vi "Report.vi"() -> ()   [LabVIEW 2017]
uses:
  <vilib>/Utility/miscctls.llb/LVRowAndColumnUnsignedTypeDef.ctl
  <vilib>/addons/database/Connection.llb/DB Tools Open Connec (String).vi
  <vilib>/Utility/file.llb/Write Delimited Spreadsheet (string).vi
  Global/Global 1.vi
  <vilib>/addons/database/NI_Database_API.lvlib
  <vilib>/Utility/NIReport.llb/NI_report.lvclass
  <vilib>/Utility/NIReport.llb/Append Text Table to Report (wrap).vi
panel:
  out "reposr save header":string[](array[string])
  out "subarray":string[](array[string])
  in  "SELECT REPORT TYPE":string(combo)="WITHOUT TRECIABILITY"
  out "error out":errorcluster
  in  "error in (no error)":errorcluster
  in  "GET REPORT":bool
  in  "EXIT":bool
  in  "EXPORT TO EXCEL":bool
  in  "TO":timestamp format="%<%x>T"
  in  "FROM":timestamp format="%<%x>T"
  in  "BARCODE":string
  in  "TYPE":string(combo)="DATE TIME"
  in  "STATION WISE":string(combo)="OP 10&20"
  out "Table":string[][](table)=[["16-06-2021 10:47:08", "A", "0.00", "0.00", "0.00", "2.03", "112.72", "3.22", "655.04", "OK"], ["16-06-2021 10:59:02", "A", "0.00", "0.00", "0.00", "0.00", "0.00", "3.02", "0.25", "NOK"]]
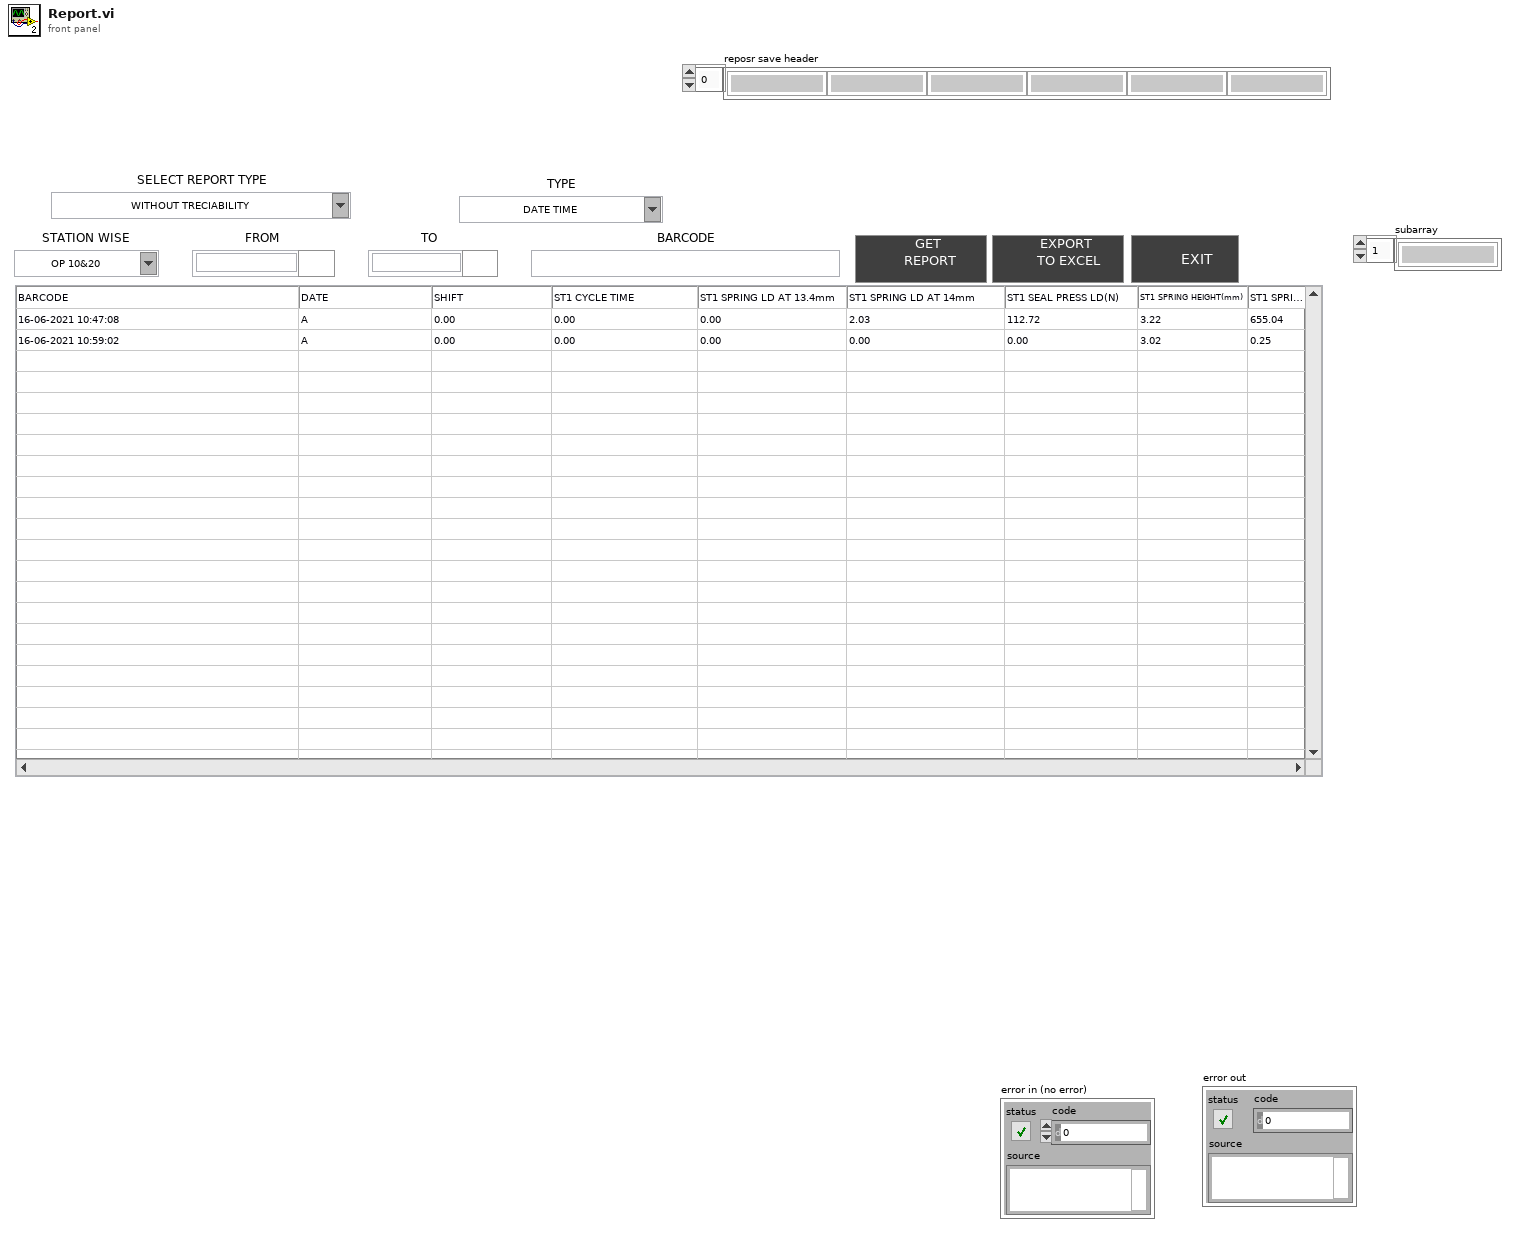
[diagram p1: front panel]
types:
  T1 = typedef "NI_Database_API.lvlib/Conn ObjectReference.ctl" = refnum<k1>
  T2 = typedef "LVRowAndColumnUnsignedTypeDef.ctl" = cluster{"Row":u32, "Column":u32}
  T3 = enum16{"Standard Report", "HTML", "Word", "Excel"}
  T4 = enum16{"maximized", "minimized", "normal", "no change"}
  T5 = enum32{"invalid app kind", "Development System", "Run Time System", "Student Edition", "Embedded LabVIEW", "Evaluation", "Custom"}
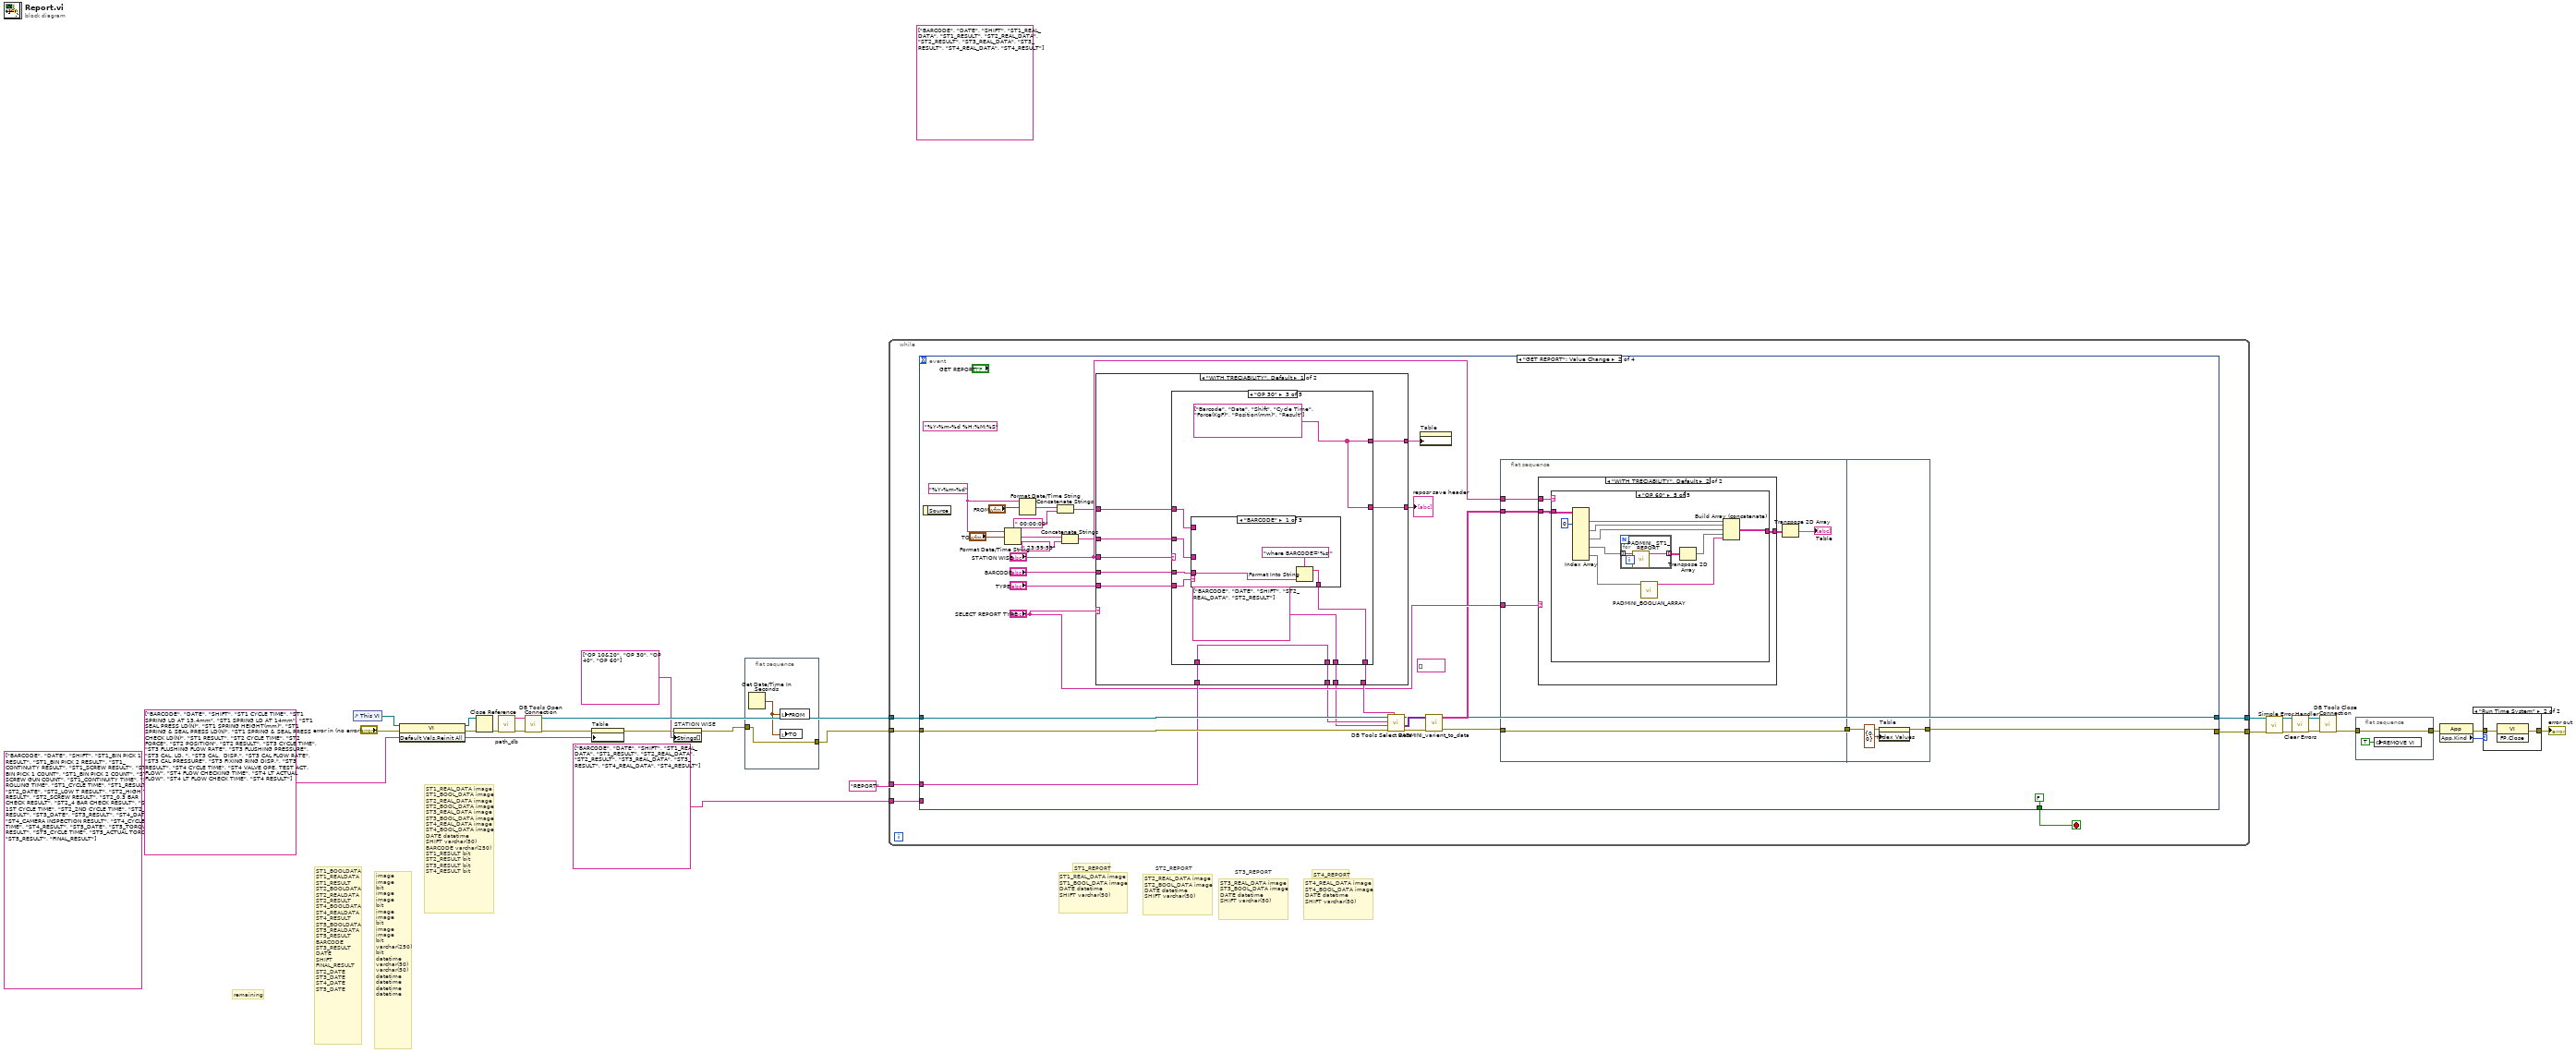
[diagram p0: block diagram]
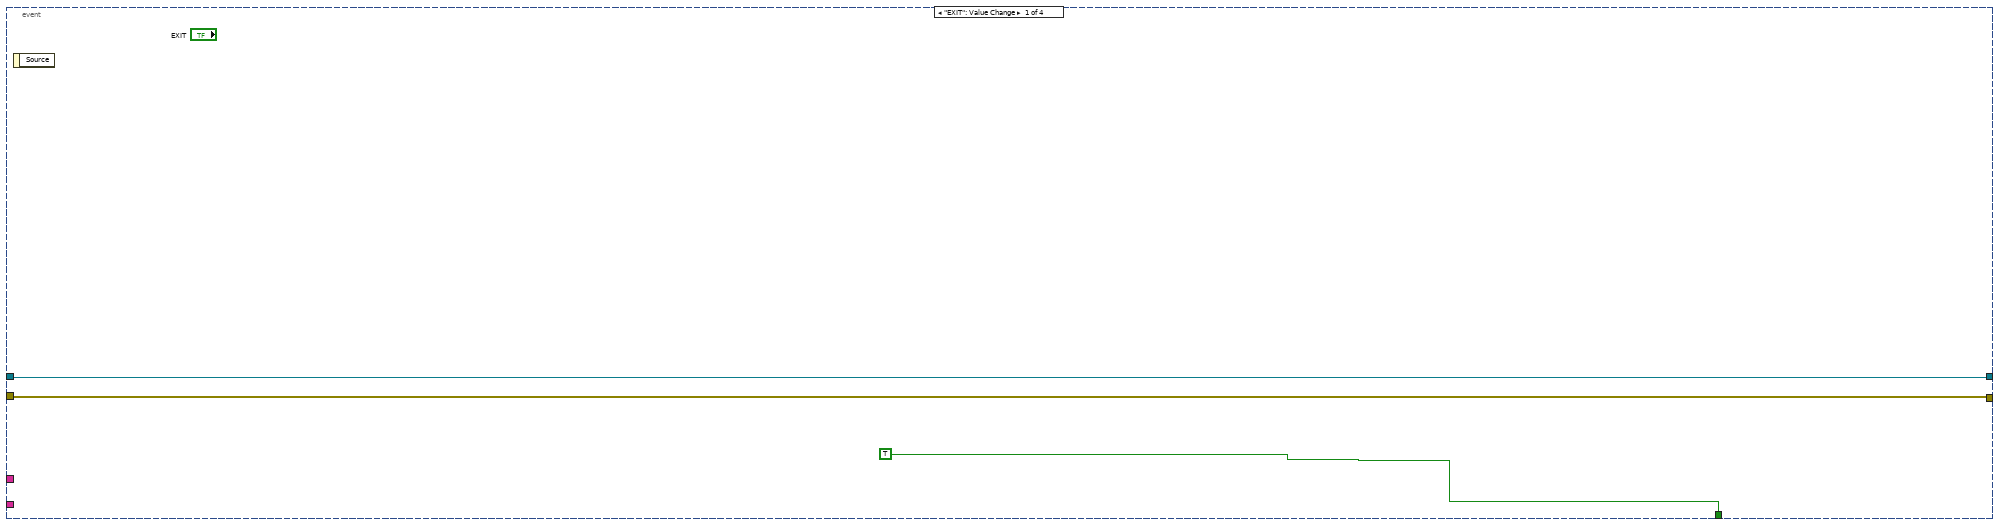
[diagram p2: hidden frame]
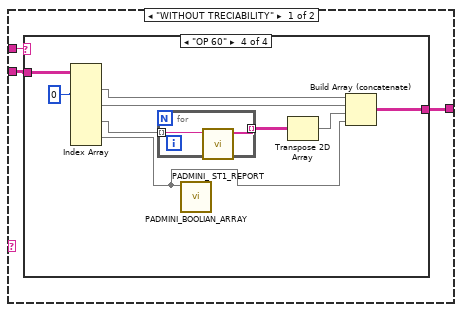
[diagram p3: hidden frame]
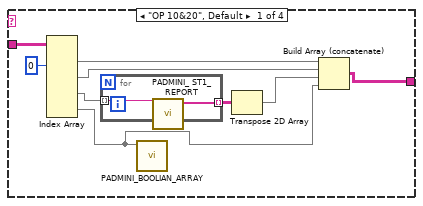
[diagram p4: hidden frame]
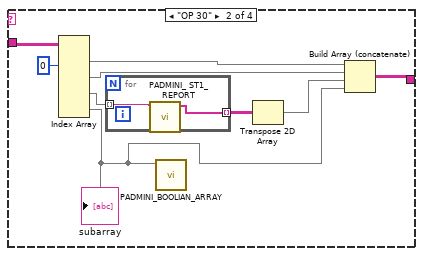
[diagram p5: hidden frame]
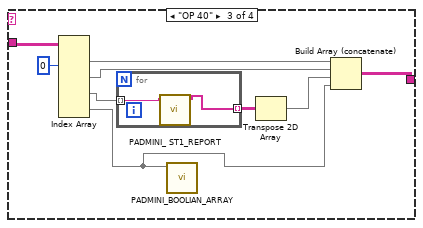
[diagram p6: hidden frame]
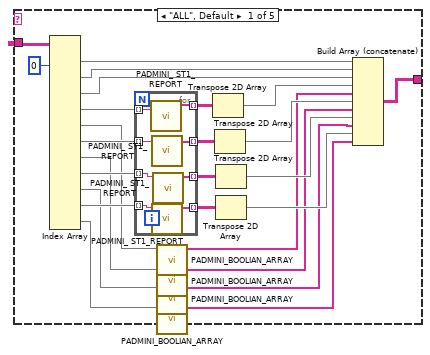
[diagram p7: hidden frame]
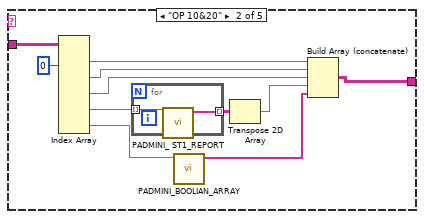
[diagram p8: hidden frame]
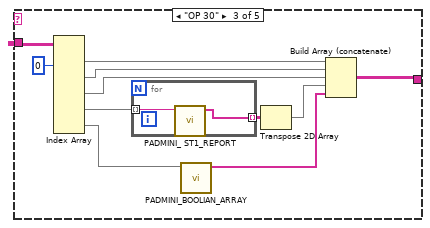
[diagram p9: hidden frame]
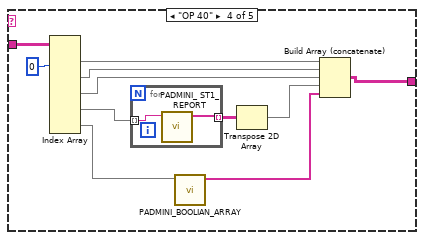
[diagram p10: hidden frame]
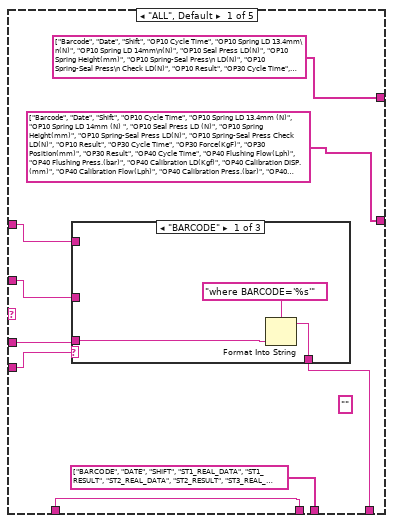
[diagram p11: hidden frame]
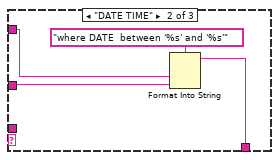
[diagram p12: hidden frame]
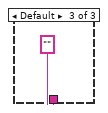
[diagram p13: hidden frame]
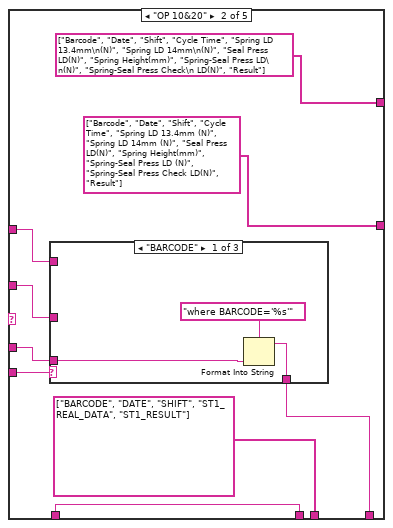
[diagram p14: hidden frame]
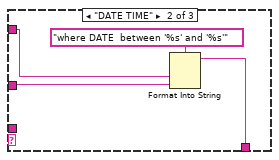
[diagram p15: hidden frame]
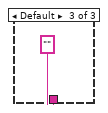
[diagram p16: hidden frame]
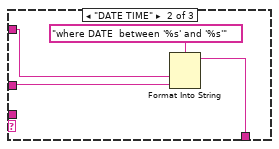
[diagram p17: hidden frame]
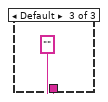
[diagram p18: hidden frame]
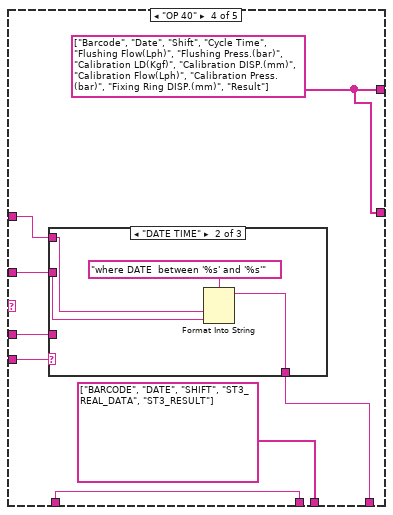
[diagram p19: hidden frame]
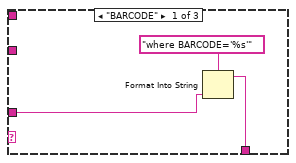
[diagram p20: hidden frame]
diagram:
  (unwired) string[] ["BARCODE", "DATE", "SHIFT", "ST1_REAL_DATA", "ST1_RESULT", "ST2_REAL_DATA", "ST2_RESULT", "ST3_REAL_DATA", "ST3_RESULT", "ST4_REAL_DATA", "ST4_RESULT"]
  (unwired) string[] ["BARCODE", "DATE", "SHIFT", "ST1_BIN PICK 1 RESULT", "ST1_BIN PICK 2 RESULT", "ST1_CONTINUITY RESULT", "ST1_SCREW RESULT", "ST1_BIN PICK 1 COUNT", "ST1_BIN PICK 2 COUNT", "ST1_SCREW GUN COUNT", "ST1_CONTINUITY TIME", "ST1_ROLLING TIME", "ST1_CYCLE TIME", "ST1_RESULT", "ST2_DATE", "ST2_LOW T RESULT", "ST2_HIGH T RESULT", "ST2_SCREW RESULT", "ST2_0.3 BAR CHECK RESULT", "ST2_4 BAR CHECK RESULT", "ST2_1ST CYCLE TIME", "ST2_2ND CYCLE TIME", "ST2_RESULT", "ST3_DATE", "ST3_RESULT", "ST4_DATE", "ST4_CAMERA INSPECTION RESULT", "ST4_CYCLE TIME", "ST4_RESULT", "ST5_DATE", "ST5_TORQUE RESULT", "ST5_CYCLE TIME", "ST5_ACTUAL TORQUE", "ST5_RESULT", "FINAL_RESULT"]
  # "remaining"
  # "ST4_REPORT"
  # "ST3_REPORT"
  # "ST2_REPORT"
  # "ST1_REPORT"
  # "ST4_REAL_DATA\timage\nST4_BOOL_DATA\timage\nDATE\tdatetime\nSHIFT\tvarchar(50)"
  # "ST3_REAL_DATA\timage\nST3_BOOL_DATA\timage\nDATE\tdatetime\nSHIFT\tvarchar(50)"
  # "ST2_REAL_DATA\timage\nST2_BOOL_DATA\timage\nDATE\tdatetime\nSHIFT\tvarchar(50)"
  # "ST1_REAL_DATA\timage\nST1_BOOL_DATA\timage\nDATE\tdatetime\nSHIFT\tvarchar(50)"
  # "ST1_REAL_DATA\timage\nST1_BOOL_DATA\timage\nST2_REAL_DATA\timage\nST2_BOOL_DATA\timage\nST3_REAL_DATA\timage\nST3_BOOL_DATA\timage\nST4_REAL_DATA\timage\nST4_BOOL_DATA\timage\nDATE\tdatetime\nSHIFT\tvarchar(50)\nBARCODE\tvarchar(250)\nST1_RESULT\tbit\nST2_RESULT\tbit\nST3_RESULT\tbit\nST4_RESULT\tbit"
  # "image\nimage\nbit\nimage\nimage\nbit\nimage\nimage\nbit\nimage\nimage\nbit\nvarchar(250)\nbit\ndatetime\nvarchar(50)\nvarchar(50)\ndatetime\ndatetime\ndatetime\ndatetime"
  # "ST1_BOOLDATA\nST1_REALDATA\nST1_RESULT\nST2_BOOLDATA\nST2_REALDATA\nST2_RESULT\nST4_BOOLDATA\nST4_REALDATA\nST4_RESULT\nST5_BOOLDATA\nST5_REALDATA\nST5_RESULT\nBARCODE\nST3_RESULT\nDATE\nSHIFT\nFINAL_RESULT\nST2_DATE\nST3_DATE\nST4_DATE\nST5_DATE"
  n1 = control-ref of="This VI"() -> (w25:refnum<vi>)
  n2 = invoke class="VI" method="Default Vals.Reinit All"(reference=w25, error in="error in (no error)") -> (reference out=w23:refnum<vi>, error out=w22:errorcluster)  [unwired: 1 in, 1 out]
  n3 = Close Reference(reference=w23, error in (no error)=w22) -> (error out=w12:errorcluster)
  n4 = call "path_db.vi"("error in"=w12) -> ("error out"=w14:errorcluster, "resulting string"=w13:string)  [unwired: 9 in]
  n5 = call-poly <vilib>:"DB Tools Open Connection.vi"("error in (no error)"=w14, "connection information"=w13) -> ("error out"=w6:errorcluster, "connection reference"=w11:T1)  [unwired: 6 in]
  n6 = property on="Table" class="Tbl (strict)"(error in=w6, "Column Headers[]"=string[] ["BARCODE", "DATE", "SHIFT", "ST1 CYCLE TIME", "ST1 SPRING LD AT 13.4mm", "ST1 SPRING LD AT 14mm", "ST1 SEAL PRESS LD(N)", "ST1 SPRING HEIGHT(mm)", "ST1 SPRING & SEAL PRESS LD(N)", "ST1 SPRING & SEAL PRESS CHECK LD(N)", "ST1 RESULT", "ST2 CYCLE TIME", "ST2 FORCE", "ST2 POSITION", "ST2 RESULT", "ST3 CYCLE TIME", "ST3 FLUSHING FLOW RATE", "ST3 FLUSHING PRESSURE", "ST3 CAL. LD. ", "ST3 CAL.  DISP.", "ST3 CAL FLOW RATE", "ST3 CAL PRESSURE", "ST3 FIXING RING DISP.", "ST3 RESULT", "ST4 CYCLE TIME", "ST4 VALVE OPE. TEST ACT. FLOW", "ST4 FLOW CHECKING TIME", "ST4 LT ACTUAL FLOW", "ST4 LT FLOW CHECK TIME", "ST4 RESULT"]) -> (error out=w3:errorcluster)  [unwired: 1 in, 1 out]
  n7 = property on="STATION WISE" class="CmbBox"(error in=w3, "Strings[]"=string[] ["OP 10&20", "OP 30", "OP 40", "OP 60"] ("Strings []")) -> (error out=w2:errorcluster)  [unwired: 1 in, 1 out]
  n8 = flat-sequence {
    tunnel: w2 -> [w26]
    tunnel: [w26] -> w1
    frame #0 {
      n9 = Get Date/Time In Seconds() -> (seconds since 1Jan1904=w27:timestamp)
      n10 = local write "FROM"(w27) -> ()
      n11 = local write "TO"(w27) -> ()
    }
  }
  n12 = while {
    tunnel: [w31] -> w15
    tunnel: w1 -> [w33]
    tunnel: w11 -> [w32]
    tunnel: [w30] -> w9
    tunnel: "REPORT" -> [w29]
    tunnel: string[] ["BARCODE", "DATE", "SHIFT", "ST1_REAL_DATA", "ST1_RESULT", "ST2_REAL_DATA", "ST2_RESULT", "ST3_REAL_DATA", "ST3_RESULT", "ST4_REAL_DATA", "ST4_RESULT"] -> [w28]
    stop <- w34 stop-if-true
    n13 = event shown="[1] \"GET REPORT\": Value Change" {
      selector: _ -> [_ _ _ _]
      dyn-events: _ -> [_ _ _ _]
      timeout: _ -> [_ _ _ _]
      tunnel: [TRUE FALSE FALSE FALSE] -> w34
      tunnel: w33 -> [w35 w65 w378 w389]
      tunnel: w32 -> [w36 w66 w381 w400]
      tunnel: [w36 w39 w381 w400] -> w30
      tunnel: [w35 w45 w377 w386] -> w31
      tunnel: w29 -> [_ w56 _ _]
      tunnel: w28 -> [_ _ _ _]
      event "EXIT": Value Change {
        n14 = event-data() -> ()  [unwired: 1 in, 1 out]
      }
      event "GET REPORT": Value Change {
        (unwired) string[] []
        (unwired) "%Y-%m-%d %H:%M:%S" ("time format string (%c)")
        w61 = "%Y-%m-%d" ("time format string (%c)")
        n15 = event-data() -> ()  [unwired: 1 in, 1 out]
        n16 = Format Date/Time String(time format string (%c)=w61, seconds (now)="TO") -> (date/time string=w50:string)  [unwired: 1 in]
        n17 = Format Date/Time String(time format string (%c)=w61, seconds (now)="FROM") -> (date/time string=w53:string)  [unwired: 1 in]
        n18 = Concatenate Strings(w53, " 00:00:00" ("time format string (%c)")) -> (w52:string)
        n19 = Concatenate Strings(w50, " 23:59:59" ("time format string (%c)")) -> (w49:string)
        n20 = case shown="\"WITH TRECIABILITY\", Default" "SELECT REPORT TYPE" {
          tunnel: "TYPE" -> [w222 w316]
          tunnel: [w221 w315] -> w63
          tunnel: "BARCODE" -> [w220 w314]
          tunnel: w52 -> [w219 w313]
          tunnel: w49 -> [w218 w312]
          tunnel: [w217 w311] -> w42
          tunnel: [w216 w310] -> w58
          tunnel: "STATION WISE" -> [w215 w309]
          tunnel: [w214 w308] -> w43
          tunnel: w56 -> [w213 w307]
          tunnel: [w212 w306] -> w44
          frame "WITH TRECIABILITY", Default {
            n21 = case shown="\"OP 30\"" w215 {
              tunnel: w222 -> [w225 w248 w264 w280 w297]
              tunnel: [w226 w247 w263 w279 w296] -> w221
              tunnel: w220 -> [w224 w246 w262 w278 w295]
              tunnel: w219 -> [w228 w245 w261 w277 w294]
              tunnel: w218 -> [w227 w244 w260 w276 w293]
              tunnel: [string[] ["BARCODE", "DATE", "SHIFT", "ST1_REAL_DATA", "ST1_RESULT", "ST2_REAL_DATA", "ST2_RESULT", "ST3_REAL_DATA", "ST3_RESULT", "ST4_REAL_DATA", "ST4_RESULT"] string[] ["BARCODE", "DATE", "SHIFT", "ST1_REAL_DATA", "ST1_RESULT"] string[] ["BARCODE", "DATE", "SHIFT", "ST2_REAL_DATA", "ST2_RESULT"] string[] ["BARCODE", "DATE", "SHIFT", "ST3_REAL_DATA", "ST3_RESULT"] string[] ["BARCODE", "DATE", "SHIFT", "ST4_REAL_DATA", "ST4_RESULT"]] -> w217
              tunnel: [string[] ["Barcode", "Date", "Shift", "OP10 Cycle Time", "OP10 Spring LD 13.4mm\n(N)", "OP10 Spring LD 14mm\n(N)", "OP10 Seal Press LD(N)", "OP10 Spring Height(mm)", "OP10 Spring-Seal Press\n LD(N)", "OP10 Spring-Seal Press\n Check LD(N)", "OP10 Result", "OP30 Cycle Time", "OP30 Force(KgF)", "OP30 Position(mm)", "OP30 Result", "OP40 Cycle Time", "OP40 Flushing Flow(Lph)", "OP40 Flushing Press.(bar)", "OP40 Calibration LD(Kgf)", "OP40 Calibration DISP.(mm)", "OP40 Calibration Flow(Lph)", "OP40 Calibration Press.(bar)", "OP40 Fixing Ring DISP.(mm)", "OP40 Result", "OP60 Cycle Time", "OP60 Valve Ope. Flow(Lpm)", "OP60 Pressure (Bar)", "OP60 Leat Test Flow(Ccm)", "OP60 LT Pressure (Bar)", "OP60 Result"] string[] ["Barcode", "Date", "Shift", "Cycle Time", "Spring LD 13.4mm\n(N)", "Spring LD 14mm\n(N)", "Seal Press LD(N)", "Spring Height(mm)", "Spring-Seal Press LD\n(N)", "Spring-Seal Press Check\n LD(N)", "Result"] w257 w273 string[] ["Barcode", "Date", "Shift", "Cycle Time", "Valve Ope. Flow(Lpm)", " Pressure (Bar)", "Leat Test Flow(Ccm)", "LT Pressure (Bar)", "Result"]] -> w216
              tunnel: [w231 w242 w258 w274 w291] -> w214
              tunnel: w213 -> [w231 w242 w258 w274 w291]
              tunnel: [string[] ["Barcode", "Date", "Shift", "OP10 Cycle Time", "OP10 Spring LD 13.4mm (N)", "OP10 Spring LD 14mm (N) ", "OP10 Seal Press LD (N)", "OP10 Spring Height(mm)", "OP10 Spring-Seal Press LD(N)", "OP10 Spring-Seal Press Check LD(N)", "OP10 Result", "OP30 Cycle Time", "OP30 Force(KgF)", "OP30 Position(mm)", "OP30 Result", "OP40 Cycle Time", "OP40 Flushing Flow(Lph)", "OP40 Flushing Press.(bar)", "OP40 Calibration LD(Kgf)", "OP40 Calibration DISP.(mm)", "OP40 Calibration Flow(Lph)", "OP40 Calibration Press.(bar)", "OP40 Fixing Ring DISP.(mm)", "OP40 Result", "OP60 Cycle Time", "OP60 Valve Ope. Flow(Lpm)", "OP60 Pressure (Bar)", "OP60 Leat Test Flow(Ccm)", "OP60 LT Pressure (Bar)", "OP60 Result"] string[] ["Barcode", "Date", "Shift", "Cycle Time", "Spring LD 13.4mm (N)", "Spring LD 14mm (N)", "Seal Press LD(N)", "Spring Height(mm)", "Spring-Seal Press LD (N)", "Spring-Seal Press Check LD(N)", "Result"] w257 w273 string[] ["Barcode", "Date", "Shift", "Cycle Time", "Valve Ope. Flow(Lpm)", "Pressure (Bar)", "Leat Test Flow(Ccm)", "LT Pressure (Bar)", "Result"]] -> w212
              frame "ALL", Default {
                (unwired) ""
                n22 = case shown="\"BARCODE\"" w225 {
                  tunnel: [w233 w237 ""] -> w226
                  tunnel: w224 -> [w232 _ _]
                  tunnel: w228 -> [_ w236 _]
                  tunnel: w227 -> [_ w235 _]
                  frame "BARCODE" {
                    n23 = Format Into String(format string="where BARCODE='%s'", w232) -> (resulting string=w233:string)  [unwired: 2 in, 1 out]
                  }
                  frame "DATE TIME" {
                    n24 = Format Into String(format string="where DATE  between '%s' and '%s'", w236, w235) -> (resulting string=w237:string)  [unwired: 2 in, 1 out]
                  }
                  frame Default {
                  }
                }
              }
              frame "OP 10&20" {
                n25 = case shown="\"BARCODE\"" w248 {
                  tunnel: [w250 w254 ""] -> w247
                  tunnel: w246 -> [w249 _ _]
                  tunnel: w245 -> [_ w253 _]
                  tunnel: w244 -> [_ w252 _]
                  frame "BARCODE" {
                    n26 = Format Into String(format string="where BARCODE='%s'", w249) -> (resulting string=w250:string)  [unwired: 2 in, 1 out]
                  }
                  frame "DATE TIME" {
                    n27 = Format Into String(format string="where DATE  between '%s' and '%s'", w253, w252) -> (resulting string=w254:string)  [unwired: 2 in, 1 out]
                  }
                  frame Default {
                  }
                }
              }
              frame "OP 30" {
                w257 = string[] ["Barcode", "Date", "Shift", "Cycle Time", "Force(KgF)", "Position(mm)", "Result"]
                n28 = case shown="\"BARCODE\"" w264 {
                  tunnel: [w266 w270 ""] -> w263
                  tunnel: w262 -> [w265 _ _]
                  tunnel: w261 -> [_ w269 _]
                  tunnel: w260 -> [_ w268 _]
                  frame "BARCODE" {
                    n29 = Format Into String(format string="where BARCODE='%s'", w265) -> (resulting string=w266:string)  [unwired: 2 in, 1 out]
                  }
                  frame "DATE TIME" {
                    n30 = Format Into String(format string="where DATE  between '%s' and '%s'", w269, w268) -> (resulting string=w270:string)  [unwired: 2 in, 1 out]
                  }
                  frame Default {
                  }
                }
              }
              frame "OP 40" {
                w273 = string[] ["Barcode", "Date", "Shift", "Cycle Time", "Flushing Flow(Lph)", "Flushing Press.(bar)", "Calibration LD(Kgf)", "Calibration DISP.(mm)", "Calibration Flow(Lph)", "Calibration Press.(bar)", "Fixing Ring DISP.(mm)", "Result"]
                n31 = case shown="\"DATE TIME\"" w280 {
                  tunnel: [w282 w286 ""] -> w279
                  tunnel: w278 -> [w281 _ _]
                  tunnel: w277 -> [_ w285 _]
                  tunnel: w276 -> [_ w284 _]
                  frame "BARCODE" {
                    n32 = Format Into String(format string="where BARCODE='%s'", w281) -> (resulting string=w282:string)  [unwired: 2 in, 1 out]
                  }
                  frame "DATE TIME" {
                    n33 = Format Into String(format string="where DATE  between '%s' and '%s'", w285, w284) -> (resulting string=w286:string)  [unwired: 2 in, 1 out]
                  }
                  frame Default {
                  }
                }
              }
              frame "OP 60" {
                n34 = case shown="\"DATE TIME\"" w297 {
                  tunnel: [w299 w303 ""] -> w296
                  tunnel: w295 -> [w298 _ _]
                  tunnel: w294 -> [_ w302 _]
                  tunnel: w293 -> [_ w301 _]
                  frame "BARCODE" {
                    n35 = Format Into String(format string="where BARCODE='%s'", w298) -> (resulting string=w299:string)  [unwired: 2 in, 1 out]
                  }
                  frame "DATE TIME" {
                    n36 = Format Into String(format string="where DATE  between '%s' and '%s'", w302, w301) -> (resulting string=w303:string)  [unwired: 2 in, 1 out]
                  }
                  frame Default {
                  }
                }
              }
            }
          }
          frame "WITHOUT TRECIABILITY" {
            n37 = case shown="\"OP 30\"" w309 {
              tunnel: w316 -> [w325 w338 w354 w367]
              tunnel: [w324 w337 w353 w366] -> w315
              tunnel: w314 -> [w323 w336 w352 w365]
              tunnel: w313 -> [w322 w335 w351 w364]
              tunnel: w312 -> [w321 w334 w350 w363]
              tunnel: [string[] ["DATE", "SHIFT", "ST1_REAL_DATA", "RESULT"] ("columns") string[] ["DATE", "SHIFT", "ST2_REAL_DATA", "RESULT"] string[] ["DATE", "SHIFT", "ST3_REAL_DATA", "RESULT"] string[] ["DATE", "SHIFT", "ST4_REAL_DATA", "RESULT"]] -> w311
              tunnel: [string[] ["Date", "Shift", "Cycle Time", "Spring LD 13.4mm\n(N)", "Spring LD 14mm\n(N)", "Seal Press LD(N)", "Spring Height(mm)", "Spring-Seal Press LD(N)", "Spring-Seal Press Check\n LD(N)", "Result"] w331 w347 w360] -> w310
              tunnel: ["ST1_REPORT" "ST2_REPORT" ("table") "ST3_REPORT" ("table") "ST4_REPORT" ("table")] -> w308
              tunnel: w307 -> [_ _ _ _]
              tunnel: [string[] ["Date", "Shift", "Cycle Time", "Spring LD 13.4mm (N)", "Spring LD 14mm (N)", "Seal Press LD(N)", "Spring Height(mm)", "Spring-Seal Press LD(N)", "Spring-Seal Press Check LD(N)", "Result"] w331 w347 w360] -> w306
              frame "OP 10&20", Default {
                # "ST1_BOOL_DATA"
                n38 = case shown="\"DATE TIME\"" w325 {
                  tunnel: [w329 ""] -> w324
                  tunnel: w323 -> [_ _]
                  tunnel: w322 -> [w328 _]
                  tunnel: w321 -> [w327 _]
                  frame "DATE TIME" {
                    n39 = Format Into String(format string="where DATE  between '%s' and '%s' order by DATE asc ", w328, w327) -> (resulting string=w329:string)  [unwired: 2 in, 1 out]
                  }
                  frame Default {
                  }
                }
              }
              frame "OP 30" {
                w331 = string[] ["Date", "Shift", "Cycle Time", "Force(KgF)", "Position(mm)", "Result"]
                n40 = case shown="\"BARCODE\"" w338 {
                  tunnel: [w340 w344 ""] -> w337
                  tunnel: w336 -> [w339 _ _]
                  tunnel: w335 -> [_ w343 _]
                  tunnel: w334 -> [_ w342 _]
                  frame "BARCODE" {
                    n41 = Format Into String(format string="where BARCODE='%s'", w339) -> (resulting string=w340:string)  [unwired: 2 in, 1 out]
                  }
                  frame "DATE TIME" {
                    n42 = Format Into String(format string="where DATE  between '%s' and '%s' order by DATE asc ", w343, w342) -> (resulting string=w344:string)  [unwired: 2 in, 1 out]
                  }
                  frame Default {
                  }
                }
              }
              frame "OP 40" {
                w347 = string[] ["Date", "Shift", "Cycle Time", "Flushing Flow(KgF)", "Flushing Press.(bar)", "Calibration LD(KgF)", "Calibration DISP.(mm)", "Calibration Flow(Lph)", "Calibration Press.(bar)", "Fixing Ring DISP.(mm)", "Result"]
                n43 = case shown="\"DATE TIME\"" w354 {
                  tunnel: [w358 ""] -> w353
                  tunnel: w352 -> [_ _]
                  tunnel: w351 -> [w357 _]
                  tunnel: w350 -> [w356 _]
                  frame "DATE TIME" {
                    n44 = Format Into String(format string="where DATE  between '%s' and '%s' order by DATE asc ", w357, w356) -> (resulting string=w358:string)  [unwired: 2 in, 1 out]
                  }
                  frame Default {
                  }
                }
              }
              frame "OP 60" {
                (unwired) string[] ["Date", "Shift", "Cycle Time", "Valve Ope. Flow(Lpm)", " Pressure (Bar)", "Leat Test Flow(Ccm)", "LT  Pressure (Bar)", "Result"]
                w360 = string[] ["Date", "Shift", "Cycle Time", "Valve Ope. Flow(Lpm)", " Pressure (Bar)", "Leat Test Flow(Ccm)", "LT  Pressure (Bar)", "Result"]
                n45 = case shown="Default" w367 {
                  tunnel: [w369 w374 ""] -> w366
                  tunnel: w365 -> [w368 _ _]
                  tunnel: w364 -> [_ w373 _]
                  tunnel: w363 -> [_ w372 _]
                  frame "BARCODE" {
                    n46 = Format Into String(format string="where BARCODE='%s'", w368) -> (resulting string=w369:string)  [unwired: 2 in, 1 out]
                  }
                  frame "DATE TIME" {
                    n47 = Format Into String(format string="where DATE  between '%s' and '%s' order by DATE asc ", w373, w372) -> (resulting string=w374:string)  [unwired: 2 in, 1 out]
                  }
                  frame Default {
                  }
                }
              }
            }
          }
        }
        "reposr save header" <- w44
        n48 = call <vilib>:"DB Tools Select Data.vi"("condition"=w63, "error in (no error)"=w65, "columns"=w42, "table"=w43, "connection reference"=w66) -> ("error out"=w48:errorcluster, "data"=w47:variant[][], "connection reference out"=w39:T1)  [unwired: 1 in]
        n49 = property on="Table" class="Tbl (strict)"("Column Headers[]"=w58) -> ()  [unwired: 2 in, 2 out]
        n50 = call "PADMINI_varient_to_data.vi"("error in (no error)"=w48, "data"=w47) -> ("error out"=w40:errorcluster, "Array"=w41:string[][])  [unwired: 8 in]
        n51 = flat-sequence {
          tunnel: "STATION WISE" -> [w72]
          tunnel: w41 -> [w71]
          tunnel: "SELECT REPORT TYPE" -> [w70]
          tunnel: w40 -> [w68]
          tunnel: [w68] -> w46
          tunnel: [w210] -> w45
          tunnel: w46 -> [w211]
          frame #0 {
            n52 = case shown="\"WITH TRECIABILITY\", Default" w70 {
              tunnel: w72 -> [w75 w122]
              tunnel: w71 -> [w74 w121]
              tunnel: [w73 w120] -> w69
              frame "WITHOUT TRECIABILITY" {
                n53 = case shown="\"OP 60\"" w75 {
                  tunnel: w74 -> [w84 w92 w103 w115]
                  tunnel: [w80 w91 w102 w114] -> w73
                  frame "OP 10&20", Default {
                    n54 = Index Array(array=w84, index (col) #1=0 ("disabled index (col)")) -> (element #1=w83:string[], element #2=w82:string[], element #3=w79:string[], element #4=w76:string[])  [unwired: 7 in]
                    n55 = for {
                      tunnel: w79 -> [w86] mode=indexing
                      tunnel: [w85] -> w78 mode=indexing
                      n56 = call "PADMINI_ ST1_REPORT.vi"("String"=w86) -> ("appended array"=w85:string[])  [unwired: 10 in]
                    }
                    n57 = call "PADMINI_BOOLIAN_ARRAY.vi"("Array in"=w76) -> ()  [unwired: 10 in, 1 out]
                    n58 = Transpose 2D Array(2D array=w78) -> (transposed array=w77:string[][])
                    n59 = Build Array (concatenate)(w83, w82, w77, w76) -> (w80:string[][])
                  }
                  frame "OP 30" {
                    n60 = Index Array(array=w92, index (col) #1=0 ("disabled index (col)")) -> (element #1=w95:string[], element #2=w94:string[], element #3=w89:string[], element #4=w87:string[])  [unwired: 7 in]
                    "subarray" <- w87
                    n61 = for {
                      tunnel: w89 -> [w97] mode=indexing
                      tunnel: [w96] -> w90 mode=indexing
                      n62 = call "PADMINI_ ST1_REPORT.vi"("String"=w97) -> ("appended array"=w96:string[])  [unwired: 10 in]
                    }
                    n63 = call "PADMINI_BOOLIAN_ARRAY.vi"("Array in"=w87) -> ()  [unwired: 10 in, 1 out]
                    n64 = Transpose 2D Array(2D array=w90) -> (transposed array=w88:string[][])
                    n65 = Build Array (concatenate)(w95, w94, w88, w87) -> (w91:string[][])
                  }
                  frame "OP 40" {
                    n66 = Index Array(array=w103, index (col) #1=0 ("disabled index (col)")) -> (element #1=w106:string[], element #2=w105:string[], element #3=w100:string[], element #4=w98:string[])  [unwired: 7 in]
                    n67 = for {
                      tunnel: w100 -> [w108] mode=indexing
                      tunnel: [w107] -> w101 mode=indexing
                      n68 = call "PADMINI_ ST1_REPORT.vi"("String"=w108) -> ("appended array"=w107:string[])  [unwired: 10 in]
                    }
                    n69 = call "PADMINI_BOOLIAN_ARRAY.vi"("Array in"=w98) -> ()  [unwired: 10 in, 1 out]
                    n70 = Transpose 2D Array(2D array=w101) -> (transposed array=w99:string[][])
                    n71 = Build Array (concatenate)(w106, w105, w99, w98) -> (w102:string[][])
                  }
                  frame "OP 60" {
                    n72 = Index Array(array=w115, index (col) #1=0 ("disabled index (col)")) -> (element #1=w117:string[], element #2=w116:string[], element #3=w113:string[], element #4=w109:string[])  [unwired: 7 in]
                    n73 = for {
                      tunnel: w113 -> [w119] mode=indexing
                      tunnel: [w118] -> w112 mode=indexing
                      n74 = call "PADMINI_ ST1_REPORT.vi"("String"=w119) -> ("appended array"=w118:string[])  [unwired: 10 in]
                    }
                    n75 = call "PADMINI_BOOLIAN_ARRAY.vi"("Array in"=w109) -> ()  [unwired: 10 in, 1 out]
                    n76 = Transpose 2D Array(2D array=w112) -> (transposed array=w110:string[][])
                    n77 = Build Array (concatenate)(w117, w116, w110, w109) -> (w114:string[][])
                  }
                }
              }
              frame "WITH TRECIABILITY", Default {
                n78 = case shown="\"OP 60\"" w122 {
                  tunnel: w121 -> [w144 w167 w174 w189 w200]
                  tunnel: [w143 w161 w173 w188 w199] -> w120
                  frame "ALL", Default {
                    n79 = Index Array(array=w144, index (col) #1=0 ("disabled index (col)")) -> (element #1=w148:string[], element #2=w147:string[], element #3=w146:string[], element #4=w142:string[], element #5=w130:string[], element #6=w137:string[], element #7=w129:string[], element #8=w136:string[], element #9=w128:string[], element #10=w135:string[], element #11=w127:string[])  [unwired: 21 in]
                    n80 = for {
                      tunnel: w142 -> [w156] mode=indexing
                      tunnel: [w155] -> w141 mode=indexing
                      tunnel: w137 -> [w154] mode=indexing
                      tunnel: [w153] -> w140 mode=indexing
                      tunnel: w136 -> [w152] mode=indexing
                      tunnel: w135 -> [w150] mode=indexing
                      tunnel: [w151] -> w134 mode=indexing
                      tunnel: [w149] -> w133 mode=indexing
                      n81 = call "PADMINI_ ST1_REPORT.vi"("String"=w156) -> ("appended array"=w155:string[])  [unwired: 10 in]
                      n82 = call "PADMINI_ ST1_REPORT.vi"("String"=w154) -> ("appended array"=w153:string[])  [unwired: 10 in]
                      n83 = call "PADMINI_ ST1_REPORT.vi"("String"=w150) -> ("appended array"=w149:string[])  [unwired: 10 in]
                      n84 = call "PADMINI_ ST1_REPORT.vi"("String"=w152) -> ("appended array"=w151:string[])  [unwired: 10 in]
                    }
                    n85 = call "PADMINI_BOOLIAN_ARRAY.vi"("Array in"=w130) -> ("Array out"=w123:string[])  [unwired: 10 in]
                    n86 = call "PADMINI_BOOLIAN_ARRAY.vi"("Array in"=w129) -> ("Array out"=w124:string[])  [unwired: 10 in]
                    n87 = call "PADMINI_BOOLIAN_ARRAY.vi"("Array in"=w128) -> ("Array out"=w125:string[])  [unwired: 10 in]
                    n88 = call "PADMINI_BOOLIAN_ARRAY.vi"("Array in"=w127) -> ("Array out"=w126:string[])  [unwired: 10 in]
                    n89 = Transpose 2D Array(2D array=w141) -> (transposed array=w139:string[][])
                    n90 = Transpose 2D Array(2D array=w140) -> (transposed array=w138:string[][])
                    n91 = Transpose 2D Array(2D array=w134) -> (transposed array=w132:string[][])
                    n92 = Transpose 2D Array(2D array=w133) -> (transposed array=w131:string[][])
                    n93 = Build Array (concatenate)(w148, w147, w146, w139, w123, w138, w124, w132, w125, w131, w126) -> (w143:string[][])
                  }
                  frame "OP 10&20" {
                    n94 = Index Array(array=w167, index (col) #1=0 ("disabled index (col)")) -> (element #1=w166:string[], element #2=w165:string[], element #3=w164:string[], element #4=w163:string[], element #5=w158:string[])  [unwired: 9 in]
                    n95 = for {
                      tunnel: w163 -> [w169] mode=indexing
                      tunnel: [w168] -> w160 mode=indexing
                      n96 = call "PADMINI_ ST1_REPORT.vi"("String"=w169) -> ("appended array"=w168:string[])  [unwired: 10 in]
                    }
                    n97 = call "PADMINI_BOOLIAN_ARRAY.vi"("Array in"=w158) -> ("Array out"=w157:string[])  [unwired: 10 in]
                    n98 = Transpose 2D Array(2D array=w160) -> (transposed array=w159:string[][])
                    n99 = Build Array (concatenate)(w166, w165, w164, w159, w157) -> (w161:string[][])
                  }
                  frame "OP 30" {
                    n100 = Index Array(array=w174, index (col) #1=0 ("disabled index (col)")) -> (element #1=w180:string[], element #2=w179:string[], element #3=w178:string[], element #4=w177:string[], element #5=w171:string[])  [unwired: 9 in]
                    n101 = for {
                      tunnel: w177 -> [w182] mode=indexing
                      tunnel: [w181] -> w176 mode=indexing
                      n102 = call "PADMINI_ ST1_REPORT.vi"("String"=w182) -> ("appended array"=w181:string[])  [unwired: 10 in]
                    }
                    n103 = call "PADMINI_BOOLIAN_ARRAY.vi"("Array in"=w171) -> ("Array out"=w170:string[])  [unwired: 10 in]
                    n104 = Transpose 2D Array(2D array=w176) -> (transposed array=w172:string[][])
                    n105 = Build Array (concatenate)(w180, w179, w178, w172, w170) -> (w173:string[][])
                  }
                  frame "OP 40" {
                    n106 = Index Array(array=w189, index (col) #1=0 ("disabled index (col)")) -> (element #1=w193:string[], element #2=w192:string[], element #3=w191:string[], element #4=w187:string[], element #5=w184:string[])  [unwired: 9 in]
                    n107 = for {
                      tunnel: w187 -> [w195] mode=indexing
                      tunnel: [w194] -> w186 mode=indexing
                      n108 = call "PADMINI_ ST1_REPORT.vi"("String"=w195) -> ("appended array"=w194:string[])  [unwired: 10 in]
                    }
                    n109 = call "PADMINI_BOOLIAN_ARRAY.vi"("Array in"=w184) -> ("Array out"=w183:string[])  [unwired: 10 in]
                    n110 = Transpose 2D Array(2D array=w186) -> (transposed array=w185:string[][])
                    n111 = Build Array (concatenate)(w193, w192, w191, w185, w183) -> (w188:string[][])
                  }
                  frame "OP 60" {
                    n112 = Index Array(array=w200, index (col) #1=0 ("disabled index (col)")) -> (element #1=w206:string[], element #2=w205:string[], element #3=w204:string[], element #4=w203:string[], element #5=w197:string[])  [unwired: 9 in]
                    n113 = for {
                      tunnel: w203 -> [w208] mode=indexing
                      tunnel: [w207] -> w202 mode=indexing
                      n114 = call "PADMINI_ ST1_REPORT.vi"("String"=w208) -> ("appended array"=w207:string[])  [unwired: 10 in]
                    }
                    n115 = call "PADMINI_BOOLIAN_ARRAY.vi"("Array in"=w197) -> ("Array out"=w196:string[])  [unwired: 10 in]
                    n116 = Transpose 2D Array(2D array=w202) -> (transposed array=w198:string[][])
                    n117 = Build Array (concatenate)(w206, w205, w204, w198, w196) -> (w199:string[][])
                  }
                }
              }
            }
            n118 = Transpose 2D Array(2D array=w69) -> (transposed array=→"Table":string[][])
          }
          frame #1 {
            n119 = property on="Table" class="Tbl (strict)"(error in=w211, "Index Values"=T2 {"Row"=0, "Column"=0}) -> (error out=w210:errorcluster)  [unwired: 1 in, 1 out]
          }
        }
      }
      event "SELECT REPORT TYPE": Value Change {
        n120 = event-data() -> ("NewVal"=w380:string)  [unwired: 1 in]
        n121 = case shown="\"WITHOUT TRECIABILITY\", Default" w380 {
          tunnel: [string[] ["ALL", "OP 10&20", "OP 30", "OP 40", "OP 60"] ("Strings []") string[] ["OP 10&20", "OP 30", "OP 40", "OP 60"] ("Strings []")] -> w379
          frame "WITH TRECIABILITY" {
          }
          frame "WITHOUT TRECIABILITY", Default {
          }
        }
        n122 = property on="STATION WISE" class="CmbBox"(error in=w378, "Strings[]"=w379) -> (error out=w377:errorcluster)  [unwired: 1 in, 1 out]
      }
      event "EXPORT TO EXCEL": Value Change {
        n123 = event-data() -> ()  [unwired: 1 in, 6 out]
        n124 = call "File Dialog"("error in"=w389) -> ("selected path"=w398:path, "error out"=w399:errorcluster)  [unwired: 11 in, 2 out]
        n125 = local read "reposr save header"() -> (w384:string[])
        n126 = call <vilib>:"Clear Errors.vi"("error in (no error)"=w399) -> ("error out"=w392:errorcluster)  [unwired: 5 in, 1 out]
        n127 = local read "Table"() -> (w401:string[][])
        n128 = property on="Table" class="Tbl (strict)" props=["Column Headers[]"](error in=w392) -> (error out=w391:errorcluster)  [unwired: 1 in, 2 out]
        n129 = Path To String(path=w398) -> (string=w397:string)
        n130 = Concatenate Strings(w397, ".csv" ("string")) -> (w395:string)
        n131 = Build Array (concatenate)(w384, w401) -> (w393:string[][])
        n132 = String To Path(string=w395) -> (path=w394:path)
        n133 = disable-structure shown="Enabled" {
          disable-tunnel: w394 -> [w420 w421]
          disable-tunnel: [w419 w423] -> w385
          disable-tunnel: w393 -> [w418 w422]
          disable-tunnel: w391 -> [w416 w423]
          disable-tunnel: [_ w422] -> w388
          disable-tunnel: [_ w421] -> w387
          frame Enabled {
            n134 = call-poly <vilib>:"Write Delimited Spreadsheet.vi"("file path (dialog if empty)"=w420, "2D data"=w418, "error in (no error)"=w416, "delimiter (\\t)"="," ("delimiter (\\t)")) -> ("error out"=w419:errorcluster)  [unwired: 10 in, 1 out]
          }
          frame Disabled {
          }
        }
        n135 = disable-structure shown="Enabled" {
          disable-tunnel: w388 -> [w405 _]
          disable-tunnel: w387 -> [w404 _]
          disable-tunnel: [w403 w415] -> w386
          disable-tunnel: w385 -> [w402 w415]
          frame Disabled {
            n136 = call <vilib>:"New Report.vi"("window state (normal)"=T4."minimized", "report type"=T3."Excel", "error in (no error)"=w402) -> ("report out"=w412:refnum<class "NI_report.lvclass">, "error out"=w411:errorcluster)  [unwired: 11 in]
            n137 = call-poly <vilib>:"Append Table to Report.vi"("report in"=w412, "text data"=w405, "error in (no error)"=w411) -> ("report out"=w408:refnum<class "NI_report.lvclass">, "error out"=w410:errorcluster)  [unwired: 9 in, 2 out]
            n138 = call-dynamic "Save Report to File.vi"("report in"=w408, "report file path"=w404, "error in (no error)"=w410) -> ("report out"=w407:refnum<class "NI_report.lvclass">, "error out"=w409:errorcluster)  [unwired: 11 in]
            n139 = call-dynamic "Dispose Report.vi"("report in"=w407, "error in (no error)"=w409, "close report? (T)"=TRUE) -> ("error out"=w403:errorcluster)  [unwired: 12 in]
          }
          frame Enabled {
          }
        }
      }
    }
  }
  n140 = call <vilib>:"Simple Error Handler.vi"("error in (no error)"=w15) -> ("error out"=w21:errorcluster)  [unwired: 4 in, 4 out]
  n141 = call <vilib>:"Clear Errors.vi"("error in (no error)"=w21) -> ("error out"=w20:errorcluster)  [unwired: 5 in, 1 out]
  n142 = call <vilib>:"DB Tools Close Connection.vi"("error in (no error)"=w20, "connection reference"=w9) -> ("error out"=w10:errorcluster)  [unwired: 5 in]
  n143 = flat-sequence {
    tunnel: [w425] -> w19
    tunnel: w10 -> [w425]
    frame #0 {
      n144 = global write "Global 1.vi" "REMOVE VI"(TRUE ("REMOVE VI")) -> ()
    }
  }
  n145 = property class="App"(error in=w19) -> (error out=w18:errorcluster, "App.Kind"=w17:T5)  [unwired: 1 in, 1 out]
  n146 = case shown="\"Run Time System\"" w17 {
    tunnel: w18 -> [w426 w428]
    tunnel: [w426 w427] -> w16
    frame "Development System", Default {
    }
    frame "Run Time System" {
      n147 = invoke class="VI" method="FP.Close"(error in=w428) -> (error out=w427:errorcluster)  [unwired: 2 in, 2 out]
    }
  }
  "error out" <- w16
